vi "16 and 2 pulses TX 8spc.vi"(7 "reset system clock":bool, 8 "referenses":T1={"clock x2"="IO Socket\\Data Clock 2x", "Memory In"="pulse on memory", "Memory In 2"="pulse on memory 2"}, 9 "IQ_run":bool=TRUE, 10 "PDW input Valid":bool, 11 "array PDW":u64[](array[numeric])=[0, 0, 0, 0]) -> (1 "pulse TX status":T2, 2 "output valid":bool, 3 "IQ out":T3[](array[typedef]), 4 "ready for input":bool)   [LabVIEW 2021]
uses:
  <instrlib>/_niInstr/DSP/v1/Shared/Public/IQ Data.ctl
  pulse_tx_vis/CTL/mode_type.ctl
  <instrlib>/_niInstr/Basic Elements/v1/FPGA/Private/Count Up U64.vi
  <instrlib>/_niInstr/Basic Elements/v1/FPGA/Private/Count Up U32.vi
  <instrlib>/_niInstr/Basic Elements/v1/FPGA/niInstr Basic Elements v1 FPGA.lvlib
  <instrlib>/_niInstr/DSP/v1/Shared/niInstr DSP v1 Shared.lvlib
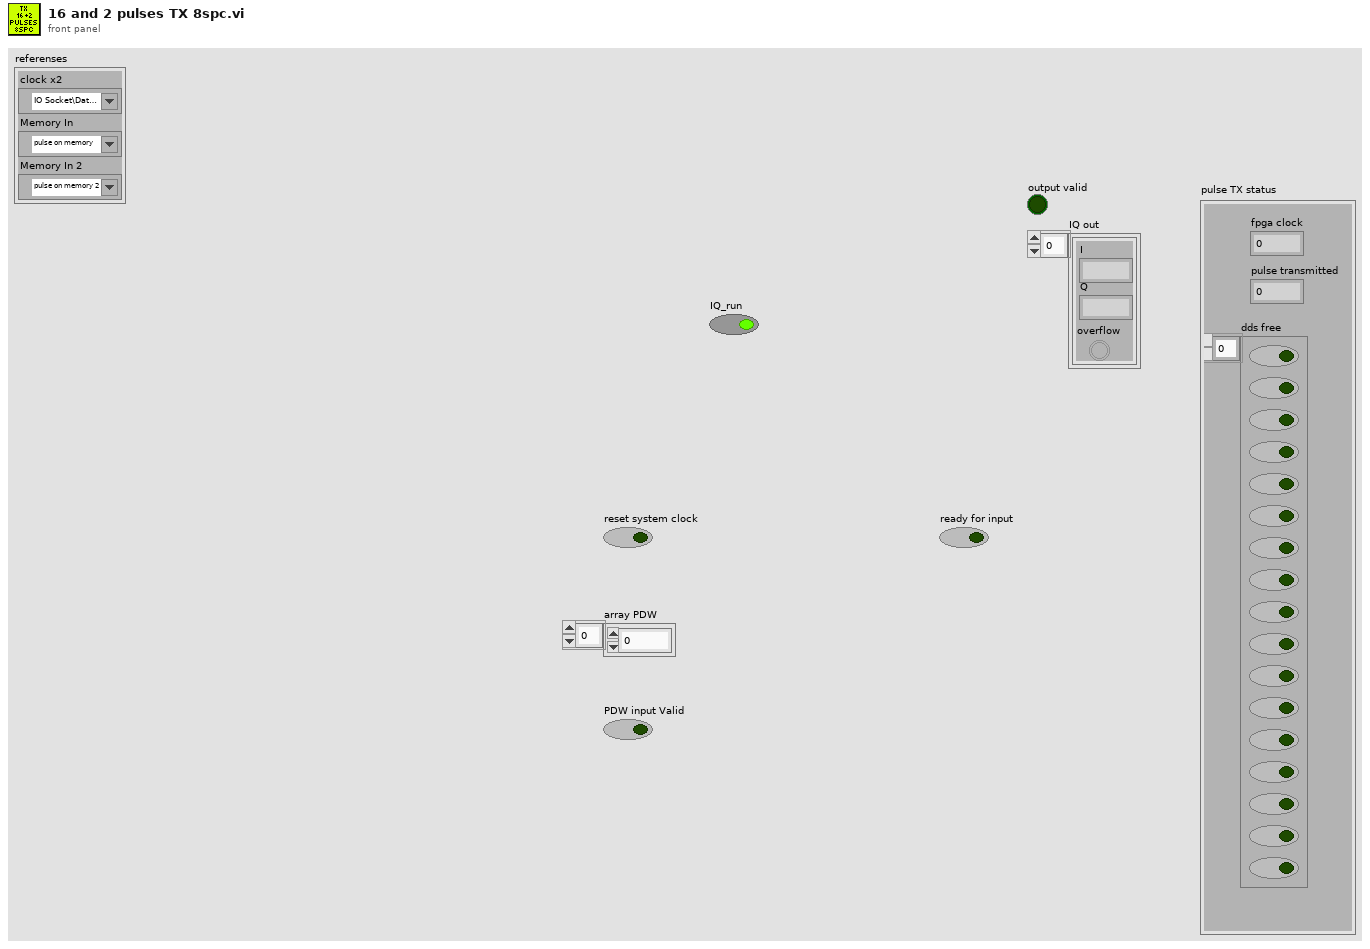
[diagram p1: front panel]
types:
  T1 = cluster{"clock x2":refnum<k21>, "Memory In":refnum<k21>, "Memory In 2":refnum<k21>}
  T2 = cluster{"fpga clock":u64, "pulse transmitted":u32, "dds free":bool[]}
  T3 = typedef "niInstr DSP v1 Shared.lvlib/IQ Data.ctl" = cluster{"I":fxp<+/-,18,1>, "Q":fxp<+/-,18,1>, "overflow":bool}
  T4 = typedef "mode_type.ctl" = enum8{"CW", "from memory 1", "NC - cw", "LFM", "BPSK", "QPSK"}
  T5 = typedef "pdw.ctl" = cluster{"PW":u32, "frequency shift":fxp<+/-,48,0>, "amp":fxp<+/-,18,1>, "mode type":T4, "mode depth":u32, "mode filter":u8, "phase shift":fxp<+/-,16,1>, "pulse shape filter":u8}
  T6 = cluster{"clock x2":refnum<k21>, "Memory In 2":refnum<k21>}
  T7 = cluster{"clock x2":refnum<k21>, "Memory In":refnum<k21>}
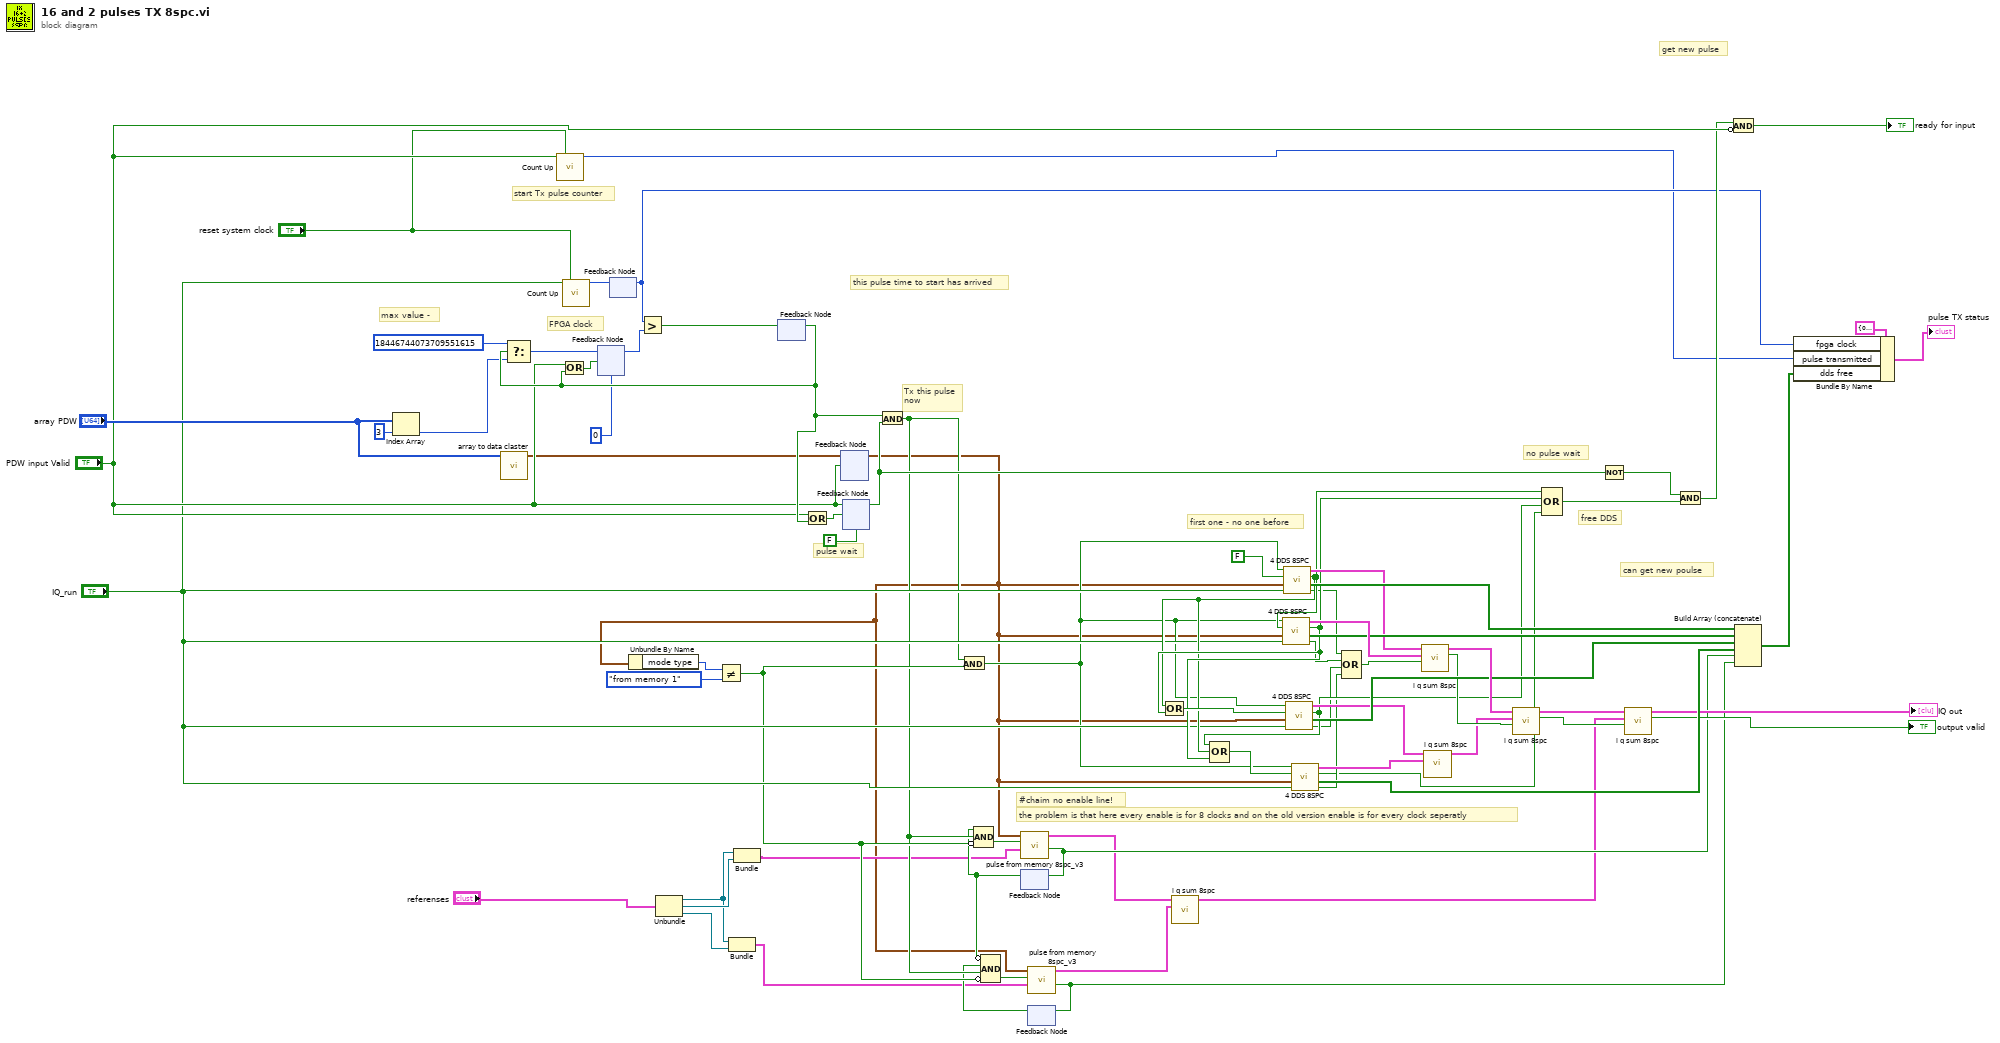
[diagram p0: block diagram]
diagram:
  # "the problem is that here every enable is for 8 clocks and on the old version enable is for every clock seperatly"
  # "#chaim no enable line!"
  # "start Tx pulse counter"
  # "FPGA clock"
  # "this pulse time to start has arrived"
  # "first one - no one before"
  # "max value -"
  # "Tx this pulse\nnow"
  # "get new pulse"
  # "pulse wait"
  # "can get new poulse"
  # "no pulse wait"
  # "free DDS"
  n1 = Index Array(array="array PDW", index=3) -> (element=w71:u64)
  n2 = call "array to data claster.vi"("Array"="array PDW") -> ("Cluster"=w25:T5)  [unwired: 10 in]
  n3 = call-poly <instrlib>:"Count Up.vi"("increment"="PDW input Valid", "reset"="reset system clock") -> ("count out"=w30:u32)  [unwired: 13 in]
  n4 = call-poly <instrlib>:"Count Up.vi"("increment"="IQ_run", "reset"="reset system clock") -> ("count out"=w64:u64)  [unwired: 13 in]
  n5 = feedback #1(u64 0 ("U64")) -> (w52:u64)
  n6 = feedback #2() -> (w31:u64)  [unwired: 1 in]
  n7 = feedback-in #2(w64) -> ()
  n8 = Greater?(x=w31, y=w52) -> (0:w74:bool)
  n9 = Unbundle("referenses") -> ("clock x2"=w6:refnum<k21>, "Memory In"=w7:refnum<k21>, "Memory In 2"=w5:refnum<k21>)
  n10 = Bundle("clock x2"=w6, "Memory In 2"=w5) -> (w4:T6)  [unwired: 1 in]
  n11 = Bundle("clock x2"=w6, "Memory In"=w7) -> (w8:T7)  [unwired: 1 in]
  n12 = feedback #3() -> (w75:bool)  [unwired: 1 in]
  n13 = Select(t=u64 18446744073709551615, s=w75, f=w71) -> (s? t:f=w57:u64)
  n14 = Or(x="PDW input Valid", y=w75) -> (x .or. y?=w58:bool)
  n15 = feedback-in #1(w57, w58) -> ()
  n16 = feedback-in #3(w74) -> ()
  n17 = Or(x="PDW input Valid", y=w75) -> (x .or. y?=w62:bool)
  n18 = feedback #4() -> (w2:T5)  [unwired: 1 in]
  n19 = Unbundle By Name(w2) -> ("mode type"=w27:T4)
  n20 = Not Equal?(x=w27, y=mode_type."from memory 1") -> (x != y?=w16:bool)
  n21 = feedback-in #4(w25, "PDW input Valid") -> ()
  n22 = feedback #5(FALSE ("Output Valid")) -> (w68:bool)
  n23 = feedback-in #5("PDW input Valid", w62) -> ()
  n24 = And(x=w75, y=w68) -> (x .and. y?=w15:bool)
  n25 = And(x=w15, y=w16) -> (x .and. y?=w24:bool)
  n26 = feedback #6() -> (w13:bool)  [unwired: 1 in]
  n27 = Compound Arithmetic op=AND(w13, w15, invert w16) -> (w23:bool)
  n28 = call "pulse from memory 8spc_v3.vi"("referenses"=w8, "start this pulse"=w23, "PDW"=w2) -> ("free DDS"=w18:bool, "IQ_out"=w12:T3[])  [unwired: 7 in]
  n29 = feedback-in #6(w18) -> ()
  n30 = feedback #7() -> (w14:bool)  [unwired: 1 in]
  n31 = Compound Arithmetic op=AND(invert w13, w14, w15, invert w16) -> (w17:bool)
  n32 = call "pulse from memory 8spc_v3.vi"("referenses"=w4, "start this pulse"=w17, "PDW"=w2) -> ("free DDS"=w3:bool, "IQ_out"=w11:T3[])  [unwired: 7 in]
  n33 = feedback-in #7(w3) -> ()
  n34 = call "i q sum 8spc.vi"("IQ in 2"=w11, "IQ in"=w12) -> ("IQ out"=w10:T3[])  [unwired: 8 in, 1 out]
  n35 = call "4 DDS 8SPC.vi"("input valid"="IQ_run", "pdw in"=w2, "free DDS before me?"=FALSE, "new PDW in"=w24) -> ("output valid"=w36:bool, "state of every DDS"=w51:bool[], "have free DDS"=w40:bool, "IQ out"=w47:T3[])  [unwired: 4 in]
  n36 = call "4 DDS 8SPC.vi"("input valid"="IQ_run", "pdw in"=w2, "free DDS before me?"=w40, "new PDW in"=w24) -> ("output valid"=w38:bool, "state of every DDS"=w50:bool[], "have free DDS"=w41:bool, "IQ out"=w69:T3[])  [unwired: 4 in]
  n37 = Or(x=w40, y=w41) -> (x .or. y?=w70:bool)
  n38 = call "4 DDS 8SPC.vi"("input valid"="IQ_run", "pdw in"=w2, "free DDS before me?"=w70, "new PDW in"=w24) -> ("output valid"=w35:bool, "state of every DDS"=w49:bool[], "have free DDS"=w39:bool, "IQ out"=w44:T3[])  [unwired: 4 in]
  n39 = Compound Arithmetic op=OR(w39, w40, w41) -> (w42:bool)
  n40 = call "4 DDS 8SPC.vi"("input valid"="IQ_run", "pdw in"=w2, "free DDS before me?"=w42, "new PDW in"=w24) -> ("output valid"=w34:bool, "state of every DDS"=w46:bool[], "have free DDS"=w1:bool, "IQ out"=w45:T3[])  [unwired: 4 in]
  n41 = Compound Arithmetic op=OR(w36, w38, w35, w34) -> (w37:bool)
  n42 = call "i q sum 8spc.vi"("input valid"=w37, "IQ in 2"=w69, "IQ in"=w47) -> ("output valid"=w48:bool, "IQ out"=w66:T3[])  [unwired: 7 in]
  n43 = call "i q sum 8spc.vi"("IQ in 2"=w45, "IQ in"=w44) -> ("IQ out"=w43:T3[])  [unwired: 8 in, 1 out]
  n44 = call "i q sum 8spc.vi"("input valid"=w48, "IQ in 2"=w43, "IQ in"=w66) -> ("output valid"=w20:bool, "IQ out"=w22:T3[])  [unwired: 7 in]
  n45 = Compound Arithmetic op=OR(w40, w41, w39, w1) -> (w65:bool)
  n46 = Not(x=w68) -> (.not. x?=w53:bool)
  n47 = call "i q sum 8spc.vi"("input valid"=w20, "IQ in 2"=w10, "IQ in"=w22) -> ("output valid"=→"output valid":bool, "IQ out"=→"IQ out":T3[])  [unwired: 7 in]
  n48 = And(x=w53, y=w65) -> (x .and. y?=w54:bool)
  n49 = Compound Arithmetic op=AND(w54, invert "PDW input Valid") -> (→"ready for input":bool)
  n50 = Build Array (concatenate)(w51, w50, w49, w46, w18, w3) -> (w29:bool[])
  n51 = Bundle By Name(cluster=T2 {"fpga clock"=0, "pulse transmitted"=0, "dds free"=[FALSE, FALSE, FALSE, FALSE, FALSE, FALSE, FALSE, FALSE, FALSE, FALSE, FALSE, FALSE, FALSE, FALSE, FALSE, FALSE, FALSE, FALSE]} ("pulse TX status"), "fpga clock"=w31, "pulse transmitted"=w30, "dds free"=w29) -> (→"pulse TX status":T2)
